vi "CDO Module to Slot Configuration.vi"(8 "error in":errorcluster, 9 "module in":refnum<class "Module.lvclass">, 10 "RSI Module in":refnum<class "RSI Module.lvclass">, 11 "slot ref in":T1 format="%.0x") -> (0 "error out":errorcluster, 3 "slot ref out":T1 format="%.0x")   [LabVIEW 2017, in "Scan Engine Scripting.lvlib"]
uses:
  Scan Engine Scripting.lvlib
  <vilib>/NI Veristand/Custom Device API/Custom Device Item Ref.ctl
  Modules.lvlibp/RSI Module/RSI Module.lvclass
  Modules/Module/Module.lvclass
  Modules.lvlibp/SD Module/SD Module.lvclass
  C:/Users/nitest/Documents/niveristand-scan-engine-ethercat-custom-device/Custom Device Source/Modules.lvlibp/RSI Module/RSI Module.lvclass
  <vilib>/NI Veristand/Custom Device API/Custom Device API.lvlib
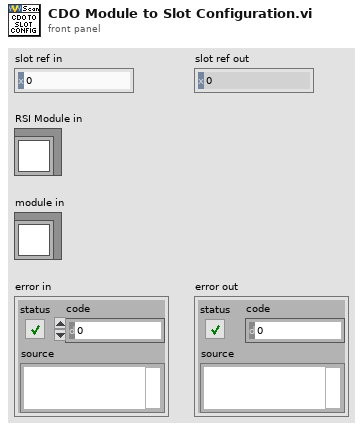
[diagram p1: front panel]
types:
  T1 = typedef "Custom Device API.lvlib/Custom Device Item Ref.ctl" = u64
  T2 = typedef "Scan Engine Scripting.lvlib/counter driven output channel settings.ctl" = cluster{"name":string, "default value":bool, "counter driven state":T3}
  T3 = typedef "Scan Engine Scripting.lvlib/Counter Driven Output Channel.lvclass/Counter Driven State.ctl" = enum16{"Disabled", "Enabled"}
  T4 = typedef "Scan Engine Scripting.lvlib/Counter Driven Output Mode.lvclass/Drive from Slot.ctl" = enum16{"Slot 1", "Slot 2", "Slot 3", "Slot 4", "Slot 5", "Slot 6", "Slot 7", "Slot 8"}
  T5 = typedef "Modules.lvlibp/SD Module.lvclass/CDO.ctl" = cluster{"Drive From Slot":u32, "CDO Channels":T6[]}
  T6 = typedef "Modules.lvlibp/SD Module.lvclass/CDO Channel.ctl" = cluster{"Counter driven enabled":bool}
  T7 = typedef "Modules.lvlibp/Custom Device API.lvlib/Custom Device Item Ref.ctl" = u64
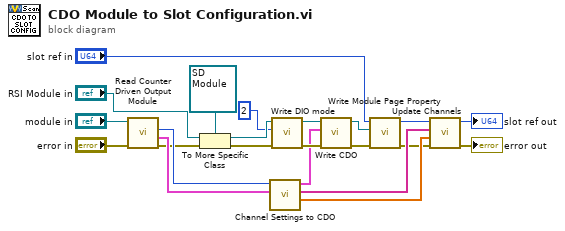
[diagram p0: block diagram]
diagram:
  n1 = call-dynamic "Read Counter Driven Output Module.vi"("error in"="error in", "module in"="module in") -> ("error out"=w4:errorcluster, "channel settings"=w14:T2[], "drive from slot"=w10:T4)  [unwired: 6 in, 1 out]
  n2 = To More Specific Class(target class=refnum<class "SD Module.lvclass"> refnum ("Modules.lvlibp:SD Module.lvclass"), reference="RSI Module in", error in=w4) -> (specific class reference=w7:refnum<class "SD Module.lvclass">, error out=w9:errorcluster)
  n3 = call "Channel Settings to CDO.vi"("channel settings"=w14, "drive from slot"=w10) -> ("channel default values"=w20:dbl[], "channel names"=w18:string[], "CDO"=w11:T5)  [unwired: 7 in]
  n4 = call-dynamic "Write DIO mode.vi"("error in (no error)"=w9, "DIO mode"=u32 2, "SD Module in"=w7) -> ("error out"=w21:errorcluster, "SD Module out"=w22:refnum<class "SD Module.lvclass">)  [unwired: 7 in]
  n5 = call-dynamic "Write CDO.vi"("error in (no error)"=w21, "CDO"=w11, "SD Module in"=w22) -> ("error out"=w12:errorcluster, "SD Module out"=w13:refnum<class "SD Module.lvclass">)  [unwired: 7 in]
  n6 = call "Write Module Page Property.vi"("error in (no error)"=w12, "RSI Module"=w13, "Node Ptr In"="slot ref in") -> ("error out"=w15:errorcluster, "Node Ptr Out"=w16:T7)  [unwired: 6 in, 1 out]
  n7 = call "Update Channels.vi"("error in"=w15, "default values"=w20, "channel names"=w18, "slot ref in"=w16) -> ("error out"=→"error out":errorcluster, "slot ref out"=→"slot ref out":T1)  [unwired: 6 in]
